vi "gRPC Client Test.vi"() -> ()   [LabVIEW 2021, in "dcvmDPI_AD7606B_client.lvlib"]
uses:
  dcvmDPI_AD7606B_client.lvlib
  dcvmDPI_AD7606B_clientImpl/dcvmDPI_AD7606B_clientImpl.lvlib
panel:
  out "Digital waveform":u32[](array[numeric])
  out "error out":errorcluster
  in  "Samples to read":u32
  in  "Input channel":i32
  in  "Digital capture samples":u32
  in  "Digital capture sample rate":dbl
  in  "Digital capture resource name":string
  in  "address":string
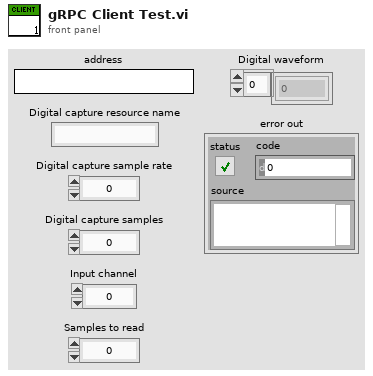
[diagram p1: front panel]
types:
  T1 = typedef "grpc-lvsupport-release.lvlib/grpcId.ctl" = u64
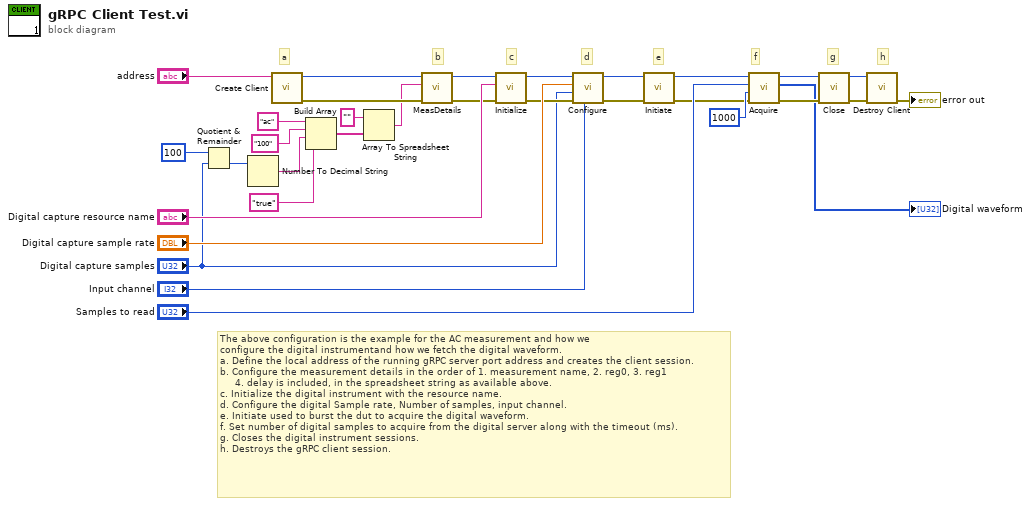
[diagram p0: block diagram]
diagram:
  # "h"
  # "g"
  # "f"
  # "e"
  # "d"
  # "c"
  # "b"
  # "a"
  # "The above configuration is the example for the AC measurement and how we \nconfigure the digital instrumentand how we fetch the digital waveform.\na. Define the local address of the running gRPC server port address and creates the client session.\nb. Configure the measurement details in the order of 1. measurement name, 2. reg0, 3. reg1\n     4. delay is included, in the spreadsheet string as available above.\nc. Initialize the digital instrument with the resource name.\nd. Configure the digital Sample rate, Number of samples, input channel.\ne. Initiate used to burst the dut to acquire the digital waveform.\nf. Set number of digital samples to acquire from the digital server along with the timeout (ms).\ng. Closes the digital instrument sessions.\nh. Destroys the gRPC client session."
  n1 = Quotient & Remainder(x=u32 100 ("y"), y="Digital capture samples") -> (floor(x/y)=w1:u32)  [unwired: 1 out]
  n2 = Number To Decimal String(number=w1) -> (decimal integer string=w4:string)  [unwired: 1 in]
  n3 = call "Create Client.vi"("address"="address") -> ("error out"=w16:errorcluster, "gRPC ID Out"=w32:T1)  [unwired: 9 in]
  n4 = Build Array("ac", "100", w4, "true") -> (w2:string[])
  n5 = Array To Spreadsheet String(array=w2, 3:"" ("format string")) -> (spreadsheet string=w9:string)  [unwired: 1 in]
  n6 = call "MeasDetails.vi"("error in"=w16, "Active measurement"=w9, "gRPC session in"=w32) -> ("error out"=w15:errorcluster, "gRPC session out"=w30:T1)  [unwired: 7 in]
  n7 = call "Initialize.vi"("error in"=w15, "Digital capture resource name"="Digital capture resource name", "gRPC session in"=w30) -> ("error out"=w14:errorcluster, "gRPC session out"=w28:T1)  [unwired: 7 in]
  n8 = call "Configure.vi"("Input channel"="Input channel", "error in"=w14, "Digital capture samples"="Digital capture samples", "Digital capture sample rate"="Digital capture sample rate", "gRPC session in"=w28) -> ("error out"=w13:errorcluster, "gRPC session out"=w25:T1)  [unwired: 5 in]
  n9 = call "Initiate.vi"("error in"=w13, "gRPC session in"=w25) -> ("error out"=w12:errorcluster, "gRPC session out"=w24:T1)  [unwired: 8 in]
  n10 = call "Acquire.vi"("error in"=w12, "Timeout (ms)"=1000, "Digital capture samples"="Samples to read", "gRPC session in"=w24) -> ("error out"=w20:errorcluster, "Digital waveform"=→"Digital waveform":u32[], "gRPC session out"=w21:T1)  [unwired: 5 in]
  n11 = call "Close.vi"("error in"=w20, "gRPC session in"=w21) -> ("error out"=w19:errorcluster, "gRPC session out"=w18:T1)  [unwired: 8 in]
  n12 = call "Destroy Client.vi"("error in"=w19, "gRPC ID"=w18) -> ("error out"=→"error out":errorcluster)  [unwired: 9 in]
